vi "Loop_Camera_acquisition.vi"() -> ()   [LabVIEW 2024, in "Camera.lvlib"]
uses:
  Camera.lvlib
  typedeff_camera_states.ctl
  typedeff_CommunicationModuleAction_Camera.ctl
  typedeff_Message_Command_Camera.ctl
  typedeff_Message_Camera.ctl
  copy_MH/Copy of Message_Handler Folder/typedeff_Message_Parameters_Camera.ctl
  <vilib>/vision/Image Controls.llb/IMAQ Image.ctl
  Message_Handler_Camera.lvlib
panel:
  out "loopCTR":u32
  out "#Frame":u32
  in  "Stop (F)":bool
  out "Live_View":T1(plugin-control)
  in  "Capture?":bool
  in  "stop":bool
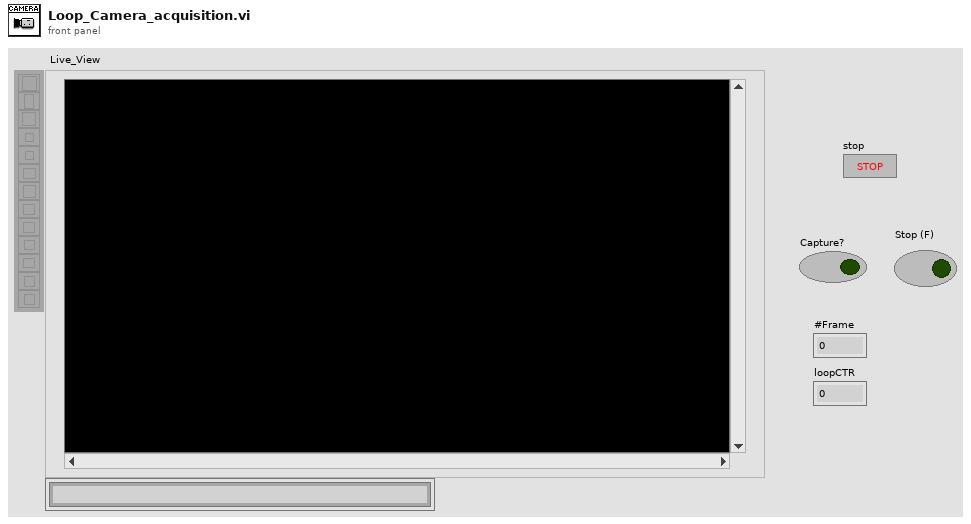
[diagram p1: front panel]
types:
  T1 = typedef "IMAQ Image.ctl" = refnum<image>
  T2 = typedef "Camera.lvlib/typedeff_camera_states.ctl" = enum16{"Error", "Init", "Idle", "Capture", "Exit", "Send_data", "Recive_Message"}
  T3 = typedef "Camera.lvlib/Message_Handler_Camera.lvlib/typedeff_CommunicationModuleAction_Camera.ctl" = enum16{"Error", "Init", "Send Msg", "Recive Msg", "Shut Down"}
  T4 = typedef "Camera.lvlib/Message_Handler_Camera.lvlib/typedeff_Message_Camera.ctl" = cluster{"Message Command":T5, "Parametr":T6}
  T5 = typedef "Camera.lvlib/Message_Handler_Camera.lvlib/typedeff_Message_Command_Camera.ctl" = enum16{"No_Message", "Send_photo"}
  T6 = typedef "Camera.lvlib/Message_Handler_Camera.lvlib/typedeff_Message_Parameters_Camera.ctl" = cluster{"Frame":T1, "Time Stamp":timestamp, "#Frame":u32}
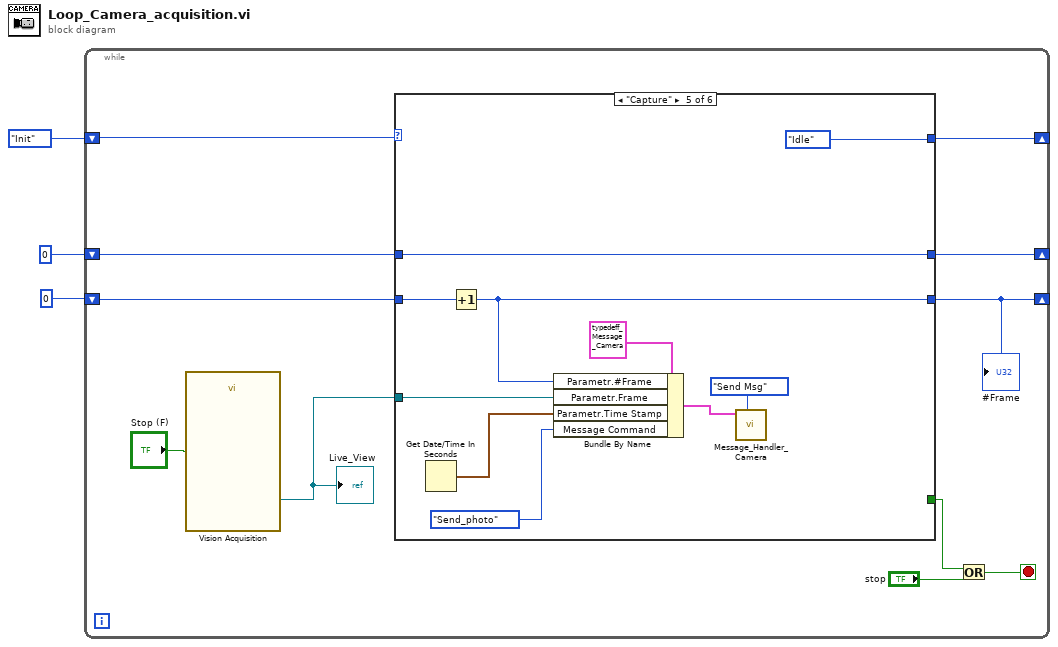
[diagram p0: block diagram]
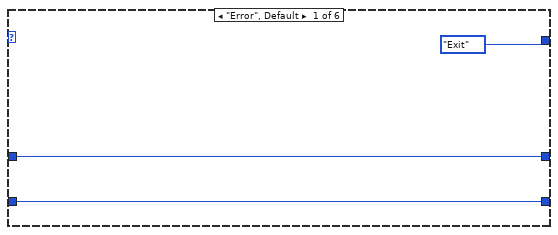
[diagram p2: hidden frame]
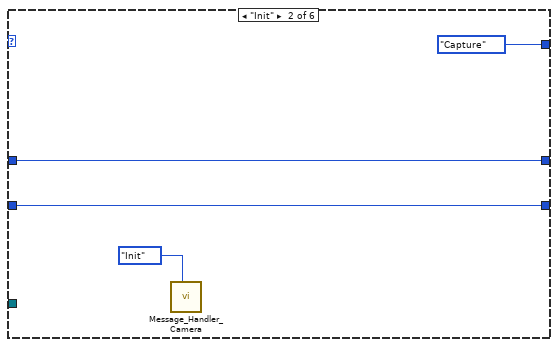
[diagram p3: hidden frame]
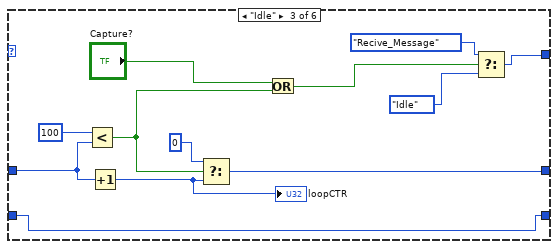
[diagram p4: hidden frame]
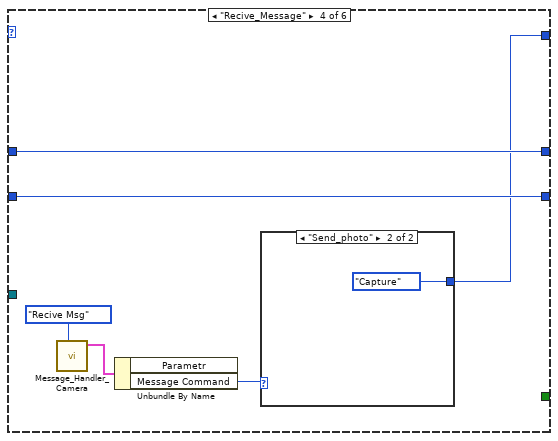
[diagram p5: hidden frame]
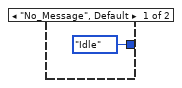
[diagram p6: hidden frame]
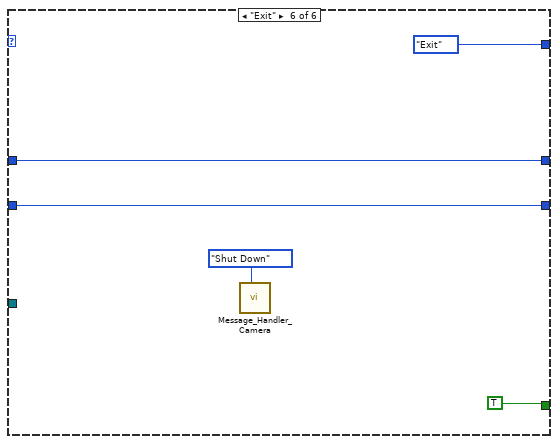
[diagram p7: hidden frame]
diagram:
  n1 = while {
    shift-right: [w13] -> _
    shift-left: u32 0 ("millisecond timer value") -> [w12]
    shift-right: [w9] -> _
    shift-left: typedeff_camera_states."Init" ("States") -> [w10]
    shift-right: [w7] -> _
    shift-left: u32 0 -> [w8]
    stop <- w4 stop-if-true
    n2 = call "Vision Acquisition"("Stop (F)"="Stop (F)") -> ("Image Out"=w11:T1)  [unwired: 24 in, 2 out]
    "Live_View" <- w11
    n3 = case shown="\"Capture\"" w10 {
      tunnel: [typedeff_camera_states."Exit" ("Cluster") typedeff_camera_states."Capture" ("States") w29 w34 typedeff_camera_states."Idle" ("States") typedeff_camera_states."Exit" ("Cluster")] -> w9
      tunnel: w11 -> [_ _ _ _ w51 _]
      tunnel: [w15 w18 w31 w38 w43 w53] -> w13
      tunnel: w12 -> [w15 w18 w26 w38 w43 w53]
      tunnel: [_ _ _ _ _ TRUE] -> w6
      tunnel: w8 -> [w16 w19 w28 w39 w45 w54]
      tunnel: [w16 w19 w28 w39 w44 w54] -> w7
      frame "Error", Default {
      }
      frame "Init" {
        n4 = call "Message_Handler_Camera.vi"("Action"=typedeff_CommunicationModuleAction_Camera."Init") -> ()  [unwired: 9 in, 2 out]
      }
      frame "Idle" {
        n5 = Less?(x=u32 100, y=w26) -> (x < y?=w24:bool)
        n6 = Increment(x=w26) -> (x+1=w27:u32)
        "loopCTR" <- w27
        n7 = Select(t=u32 0 ("x"), s=w24, f=w27) -> (s? t:f=w31:u32)
        n8 = Or(x="Capture?", y=w24) -> (x .or. y?=w32:bool)
        n9 = Select(t=typedeff_camera_states."Recive_Message" ("States"), s=w32, f=typedeff_camera_states."Idle" ("States")) -> (s? t:f=w29:T2)
      }
      frame "Recive_Message" {
        n10 = call "Message_Handler_Camera.vi"("Action"=typedeff_CommunicationModuleAction_Camera."Recive Msg") -> ("Message_OUT"=w36:T4)  [unwired: 9 in, 1 out]
        n11 = Unbundle By Name(w36) -> ("Message Command"=w35:T5)  [unwired: 1 out]
        n12 = case shown="\"Send_photo\"" w35 {
          tunnel: [typedeff_camera_states."Idle" ("States") typedeff_camera_states."Capture" ("States")] -> w34
          frame "No_Message", Default {
          }
          frame "Send_photo" {
          }
        }
      }
      frame "Capture" {
        n13 = Get Date/Time In Seconds() -> (seconds since 1Jan1904=w50:timestamp)
        n14 = Increment(x=w45) -> (x+1=w44:u32)
        n15 = Bundle By Name(cluster=T4 {"Message Command"=enum."No_Message", "Parametr"={"Frame"=refnum, "Time Stamp"=timestamp(0 s since 1904-01-01), "#Frame"=0}} ("Message"), "Parametr.#Frame"=w44, "Parametr.Frame"=w51, "Parametr.Time Stamp"=w50, "Message Command"=typedeff_Message_Command_Camera."Send_photo") -> (w47:T4)
        n16 = call "Message_Handler_Camera.vi"("Action"=typedeff_CommunicationModuleAction_Camera."Send Msg", "Message_IN"=w47) -> ()  [unwired: 8 in, 2 out]
      }
      frame "Exit" {
        n17 = call "Message_Handler_Camera.vi"("Action"=typedeff_CommunicationModuleAction_Camera."Shut Down") -> ()  [unwired: 9 in, 2 out]
      }
    }
    "#Frame" <- w7
    n18 = Or(x=w6, y="stop") -> (x .or. y?=w4:bool)
  }
